vi "导出校准基准数据.vi"(8 "error in":errorcluster, 9 "OUT":i32=4, 11 "IN":i32=128) -> (0 "error out":errorcluster)   [LabVIEW 2015]
uses:
  <vilib>/addons/_office/excel.llb/Excel Easy Table (str).vi
  server/Global/SeverGlobal.vi
  <vilib>/Utility/NIReport.llb/NI_report.lvclass
  <vilib>/Utility/NIReport.llb/Excel/NI_Excel.lvclass
  <vilib>/addons/_office/NI_ReportGenerationToolkit.lvlib
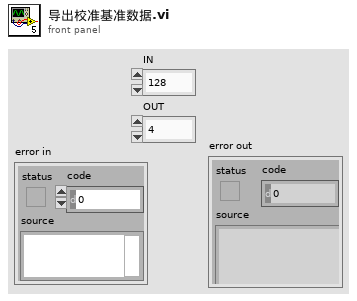
[diagram p1: front panel]
types:
  T1 = enum16{"Standard Report", "HTML", "Word", "Excel"}
  T2 = enum16{"maximized", "minimized", "normal", "no change"}
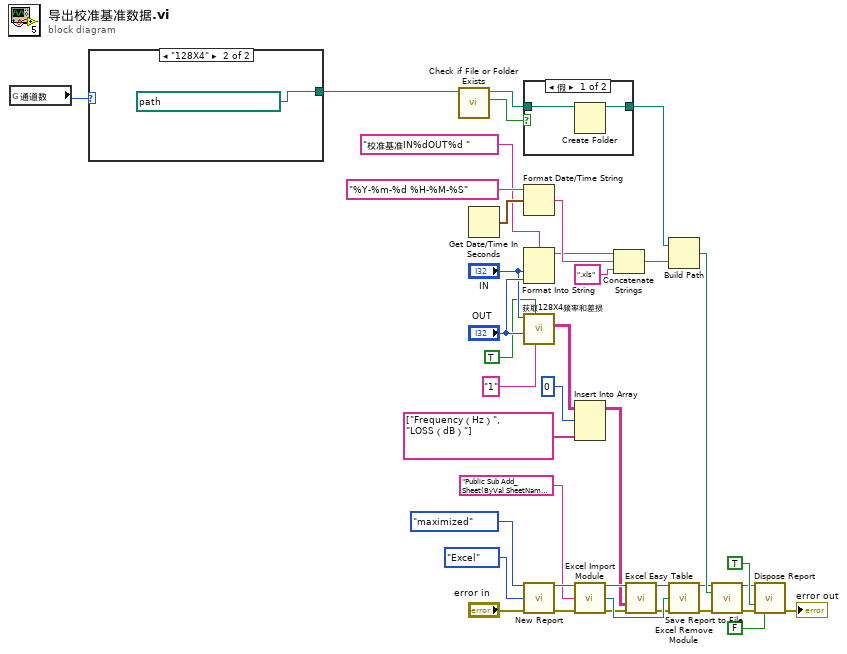
[diagram p0: block diagram]
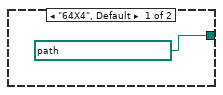
[diagram p2: hidden frame]
diagram:
  n1 = global read "SeverGlobal.vi" "通道数"() -> (w2:enum16{"64X4", "128X4"})
  n2 = case shown="\"128X4\"" w2 {
    tunnel: [path "D:/64X4数据/基准数据" ("base path") path "D:/128X4数据/基准数据" ("base path")] -> w1
    frame "64X4", Default {
    }
    frame "128X4" {
    }
  }
  n3 = call <vilib>:"Check if File or Folder Exists.vi"("path"=w1) -> ("file or folder exists?"=w21:bool, "dup path"=w20:path)  [unwired: 8 in, 1 out]
  n4 = Get Date/Time In Seconds() -> (seconds since 1Jan1904=w24:timestamp)
  n5 = case shown="假" w21 {
    tunnel: w20 -> [w43 w44]
    tunnel: [w42 w44] -> w19
    frame False {
      n6 = Create Folder(path (use dialog)=w43) -> (created path=w42:path)  [unwired: 2 in, 2 out]
    }
    frame True {
    }
  }
  n7 = Format Date/Time String(time format string (%c)="%Y-%m-%d %H-%M-%S", seconds (now)=w24) -> (date/time string=w27:string)  [unwired: 1 in]
  n8 = Format Into String(format string="校准基准IN%dOUT%d ", "IN", "OUT") -> (resulting string=w17:string)  [unwired: 2 in, 1 out]
  n9 = call "获取128X4频率和差损.vi"("testType"="1", "ref"=TRUE, "COM"="OUT", "A"="IN") -> ("Freq&S21"=w6:string[][])  [unwired: 6 in, 1 out]
  n10 = call <vilib>:"New Report.vi"("window state (normal)"=T2."maximized", "report type"=T1."Excel", "error in (no error)"="error in") -> ("report out"=w38:refnum<class "NI_report.lvclass">, "error out"=w39:errorcluster)  [unwired: 11 in]
  n11 = Insert Into Array(array=w6, index (row)=0, new element=string[] ["Frequency（Hz）", "LOSS（dB）"] ("new element/subarray")) -> (w5:string[][])  [unwired: 1 in]
  n12 = call <vilib>:"Excel Import Module.vi"("report in"=w38, "module code (\"\")"="Public Sub Add_Sheet(ByVal SheetName As String)\n    Dim shcount As Integer\n    shcount = Sheets.Count\n    Sheets.Add after:=Sheets(shcount)\n    shcount = shcount + 1\n    Sheets(shcount).Name = SheetName\nEnd Sub" ("module code (\"\")"), "error in (no error)"=w39) -> ("report out"=w12:refnum<class "NI_report.lvclass">, "module reference"=w22:refnum<k7>, "error out"=w11:errorcluster)  [unwired: 10 in]
  n13 = Concatenate Strings(w17, w27, ".xls") -> (w28:string)
  n14 = call-poly <vilib>:"Excel Easy Table.vi"("report in"=w12, "text data"=w5, "error in (no error)"=w11) -> ("report out"=w9:refnum<class "NI_report.lvclass">, "error out"=w10:errorcluster)  [unwired: 8 in, 3 out]
  n15 = Build Path(base path=w19, name or relative path=w28) -> (appended path=w23:path)
  n16 = call <vilib>:"Excel Remove Module.vi"("report in"=w9, "module reference"=w22, "error in (no error)"=w10) -> ("report out"=w4:refnum<class "NI_report.lvclass">, "error out"=w3:errorcluster)  [unwired: 11 in]
  n17 = call-dynamic "Save Report to File.vi"("report in"=w4, "report file path"=w23, "error in (no error)"=w3) -> ("report out"=w29:refnum<class "NI_report.lvclass">, "error out"=w30:errorcluster)  [unwired: 11 in]
  n18 = call-dynamic "Dispose Report.vi"("report in"=w29, "save changes? (F)"=TRUE, "error in (no error)"=w30, "close report? (T)"=FALSE) -> ("error out"=→"error out":errorcluster)  [unwired: 11 in]
